vi "build memory.vi"(8 "error in (no error)":errorcluster caption="에러 입력(에러 없음)", 10 "WF List":T1[](array[typedef]), 11 "DW7912 입력":refnum<class "DW7912.lvclass">) -> (0 "error out":errorcluster caption="에러 출력", 1 "memory data by wf":cluster{"Header":u8[], "Data":u8[]}[](array[cluster]), 2 "full memory data":u8[](array[numeric]), 3 "DW7912 출력":refnum<class "DW7912.lvclass">)   [LabVIEW 2020, in "DW7912.lvclass"]
uses:
  DW7912.lvclass
  SubVIs/Waveform Editor/Controls/(Ctrl)Waveform Editor_WF List.ctl
  Waveform Obj Class/Waveform Obj/Waveform Obj.lvclass
  Waveform Obj Class/Waveform Obj/Waveform Obj.lvclass/Waveform Obj.ctl
  Waveform Obj Class/Waveform Obj/Accessors/Read voltage range.vi
  Waveform Obj Class/Waveform Obj/Accessors/Read sampling rate.vi
  Waveform Obj Class/Waveform Obj/Accessors/Read wait.vi
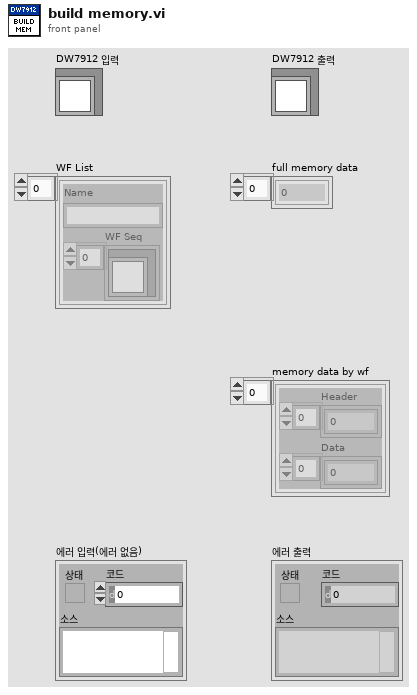
[diagram p1: front panel]
types:
  T1 = typedef "(Ctrl)Waveform Editor_WF List.ctl" = cluster{"Name":string, "WF Seq":refnum<class "Waveform Obj.lvclass">[]}
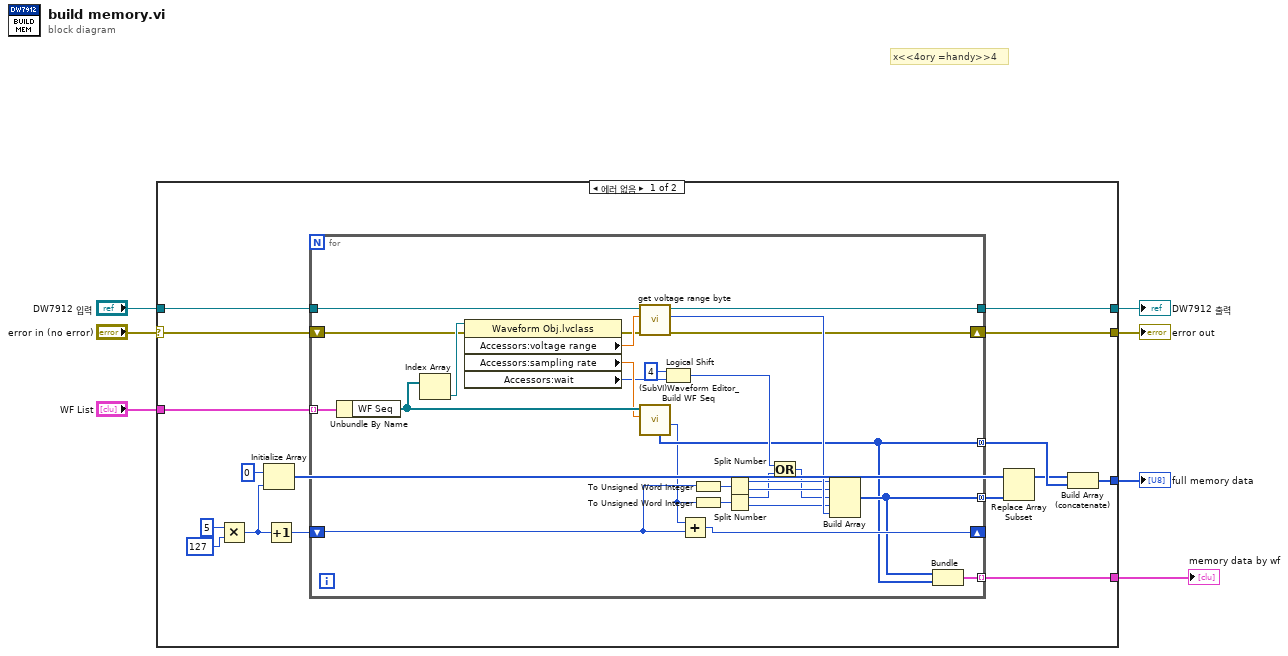
[diagram p0: block diagram]
diagram:
  # "x<<4ory =handy>>4"
  n1 = case shown="에러 없음" "error in (no error)" {
    selector: "error in (no error)" -> [w20 w51]
    tunnel: "DW7912 입력" -> [w21 w52]
    tunnel: "WF List" -> [w19 _]
    tunnel: [w18 w52] -> w4
    tunnel: [w17 w51] -> w3
    tunnel: [w16 _] -> w2
    tunnel: [w8 _] -> w1
    frame No Error {
      n2 = Multiply(x=5, y=127) -> (x*y=w12:i32)
      n3 = Initialize Array(u8 0 ("원소"), w12) -> (w10:u8[])
      n4 = Increment(x=w12) -> (x+1=w14:i32)
      n5 = for {
        tunnel: w19 -> [w49] mode=indexing
        shift-right: [w48] -> _
        shift-left: w14 -> [w34]
        tunnel: [w27] -> w22 mode=concatenating
        tunnel: w21 -> [w46]
        tunnel: [w28] -> w11 mode=concatenating
        tunnel: [w40] -> w18
        shift-right: [w39] -> w17
        shift-left: w20 -> [w36]
        tunnel: [w26] -> w8 mode=indexing
        n6 = Unbundle By Name(w49) -> ("WF Seq"=w47:refnum<class "Waveform Obj.lvclass">[])
        n7 = Index Array(array=w47) -> (element=w42:refnum<class "Waveform Obj.lvclass">)  [unwired: 1 in]
        n8 = property class="Waveform Obj.lvclass"(reference=w42, error in=w36) -> (error out=w35:errorcluster, "Accessors:voltage range"=w37:dbl, "Accessors:sampling rate"=w38:dbl, "Accessors:wait"=w33:u8)  [unwired: 1 out]
        n9 = call-dynamic "get voltage range byte.vi"("error in (no error)"=w35, "voltage range"=w37, "DW7912 입력"=w46) -> ("error out"=w39:errorcluster, "byte value"=w50:u8, "DW7912 출력"=w40:refnum<class "DW7912.lvclass">)  [unwired: 6 in]
        n10 = call "(SubVI)Waveform Editor_Build WF Seq.vi"("Sampling Rate"=w38, "WF Seq"=w47) -> ("number of wf samples"=w25:i32, "8bit memory data"=w27:u8[])  [unwired: 4 in, 4 out]
        n11 = Logical Shift(y=i16 4, x=w33) -> (x << y=w30:u8)
        n12 = Add(x=w25, y=w34) -> (x+y=w48:i32)
        n13 = To Unsigned Word Integer(number=w34) -> (unsigned 16bit integer=w44:u16)
        n14 = To Unsigned Word Integer(number=w25) -> (unsigned 16bit integer=w41:u16)
        n15 = Split Number(x=w44) -> (hi(x)=w45:u8, lo(x)=w43:u8)
        n16 = Split Number(x=w41) -> (hi(x)=w31:u8, lo(x)=w24:u8)
        n17 = Or(x=w30, y=w31) -> (x .or. y?=w29:u8)
        n18 = Build Array(w45, w43, w29, w24, w50) -> (w28:u8[])
        n19 = Bundle(w28, "8bit memory data"=w27) -> (w26:cluster{u8[], "8bit memory data":u8[]})  [unwired: 1 in]
      }
      n20 = Replace Array Subset(array=w10, new element=w11) -> (w9:u8[])  [unwired: 1 in]
      n21 = Build Array (concatenate)(w9, w22) -> (w16:u8[])
    }
    frame Error {
    }
  }
  "error out" <- w3
  "DW7912 출력" <- w4
  "full memory data" <- w2
  "memory data by wf" <- w1
